vi "test_transceiver_error_test.vi"(8 "error in (no error)":errorcluster, 11 "TestCase in":refnum<class "DSFPluginTestCase.lvclass">) -> (0 "error out":errorcluster, 3 "TestCase out":refnum<class "DSFPluginTestCase.lvclass">)   [LabVIEW 2017, in "DSFPluginTestCase.lvclass"]
uses:
  DSFPluginTestCase.lvclass
  <vilib>/addons/_JKI Toolkits/VI Tester/TestCase.llb/TestCase.lvclass
  C:/Program Files (x86)/National Instruments/LabVIEW 2017/vi.lib/addons/_JKI Toolkits/VI Tester/TestCase.llb/TestCase.lvclass
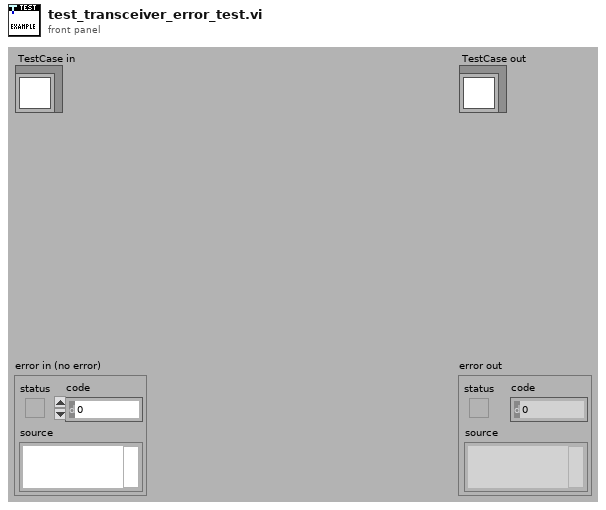
[diagram p1: front panel]
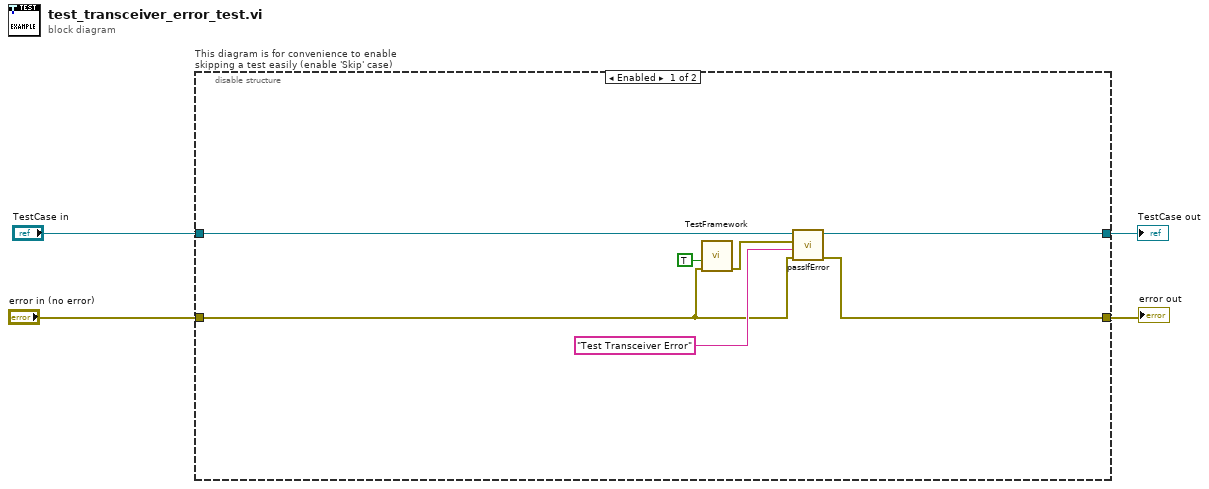
[diagram p0: block diagram]
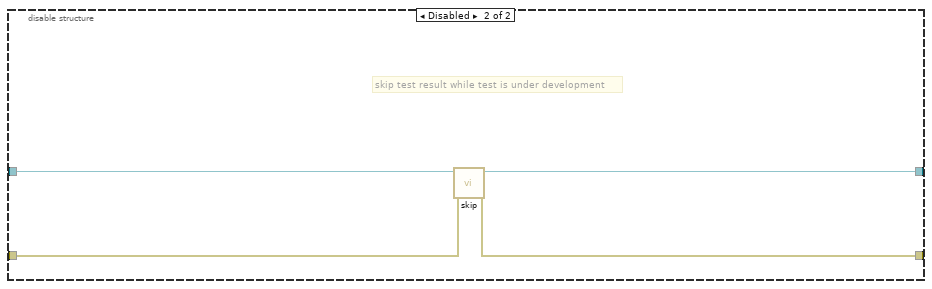
[diagram p2: hidden frame]
diagram:
  n1 = disable-structure "This diagram is for convenience to enable skipping a test easily (enable 'Skip' case)" shown="Enabled" {
    disable-tunnel: "TestCase in" -> [w7 w15]
    disable-tunnel: [w6 w13] -> w1
    disable-tunnel: [w5 w14] -> w3
    disable-tunnel: "error in (no error)" -> [w8 w12]
    frame Enabled {
      n2 = call "TestFramework.vi"("error in (no error)"=w8, "Simulate Error?"=TRUE) -> ("error out"=w10:errorcluster)  [unwired: 8 in, 1 out]
      n3 = call-dynamic "passIfError.vi"("error in (no error)"=w8, "task (\"\")"="Test Transceiver Error" ("task (\"\")"), "error"=w10, "TestCase in"=w7) -> ("error out"=w5:errorcluster, "TestCase out"=w6:refnum<class "DSFPluginTestCase.lvclass">)  [unwired: 6 in]
    }
    frame Disabled {
      # "skip test result while test is under development"
      n4 = call <vilib>:"skip.vi"("error in (no error)"=w12, "TestCase in"=w15) -> ("error out"=w14:errorcluster, "TestCase out"=w13:refnum<class "DSFPluginTestCase.lvclass">)  [unwired: 8 in]
    }
  }
  "error out" <- w3
  "TestCase out" <- w1
